vi "Save File Check Special Characters.vi"(8 "Error In":errorcluster, 11 "Filename":string) -> (0 "Error Out":errorcluster, 3 "Filename Output":string)   [LabVIEW 2019, in "Save File.lvlib"]
uses:
  Save File.lvlib
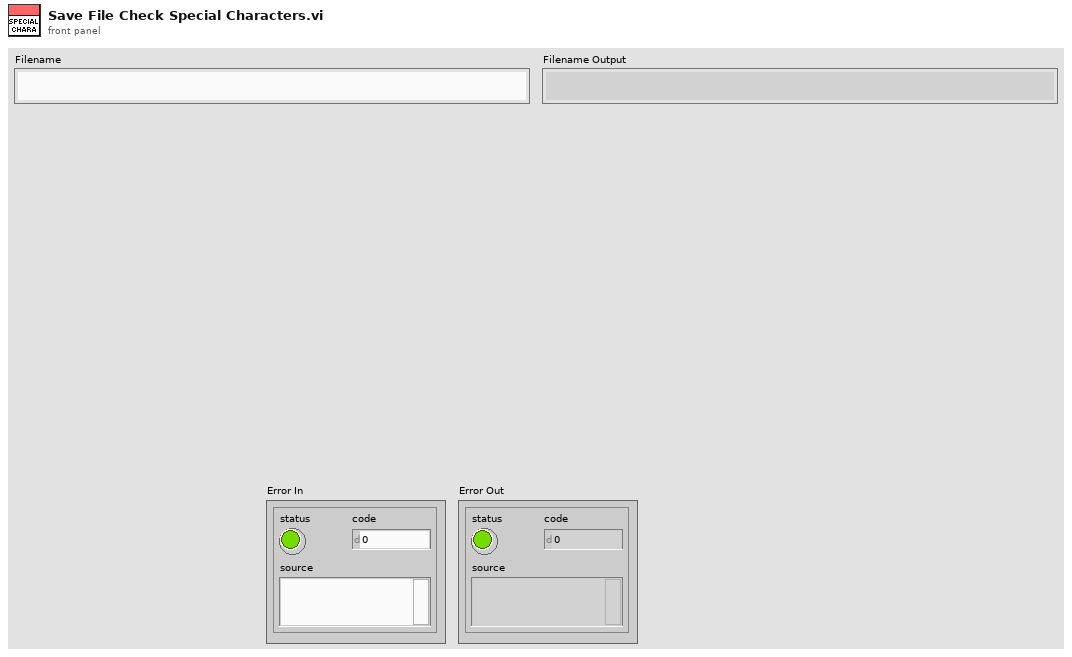
[diagram p1: front panel]
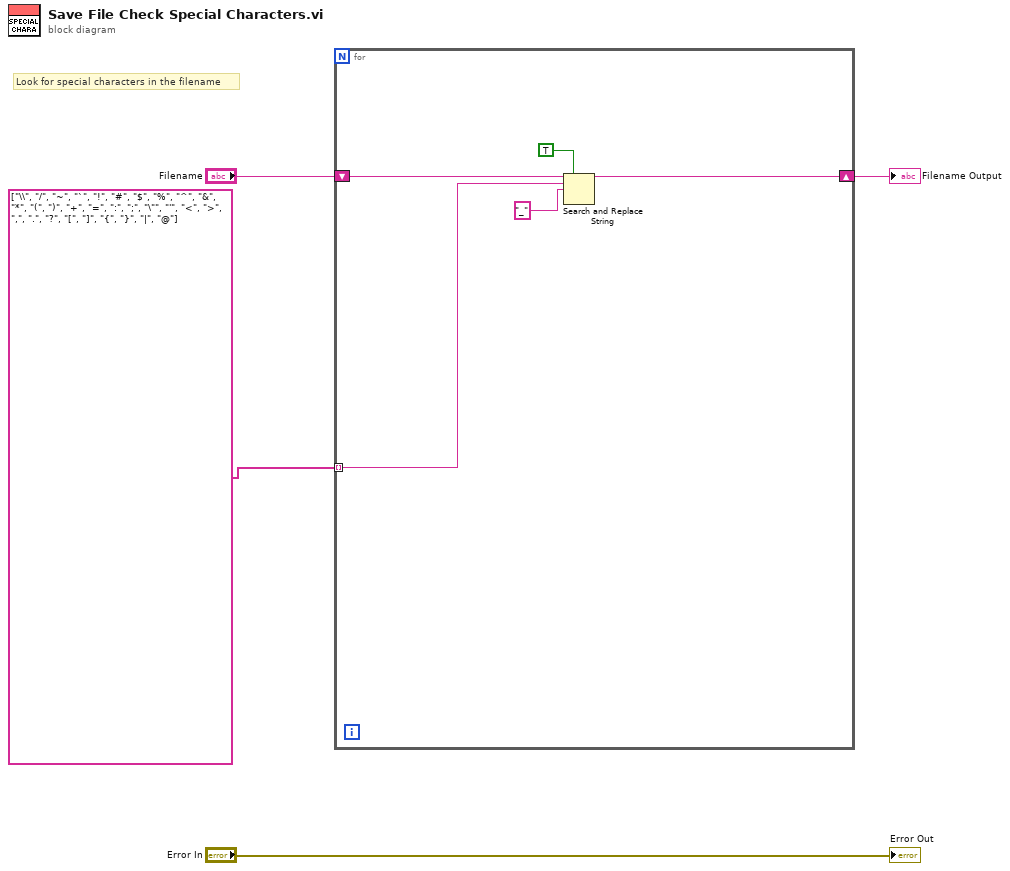
[diagram p0: block diagram]
diagram:
  # "Look for special characters in the filename"
  n1 = for {
    tunnel: string[] ["\\", "/", "~", "`", "!", "#", "$", "%", "^", "&", "*", "(", ")", "+", "=", ":", ";", "\"", "'", "<", ">", ",", ".", "?", "[", "]", "{", "}", "|", "@"] -> [w7] mode=indexing
    shift-right: [w8] -> w1
    shift-left: "Filename" -> [w9]
    n2 = Search and Replace String(replace all?=TRUE ("replace all? (F)"), input string=w9, search string=w7, replace string="_" ("string")) -> (result string=w8:string)  [unwired: 4 in, 3 out]
  }
  "Filename Output" <- w1
  "Error Out" <- "Error In"
